vi "P4CMD_Sup Expand Wildcards.vi"(4 "string input":string) -> (1 "string output":string)   [LabVIEW 2020, in "NI_SCC_P4CMD.lvlib"]
uses:
  <vilib>/SourceControl/Providers/P4CMD/NI_SCC_P4CMD.lvlib
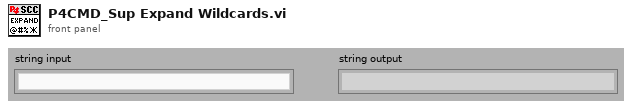
[diagram p1: front panel]
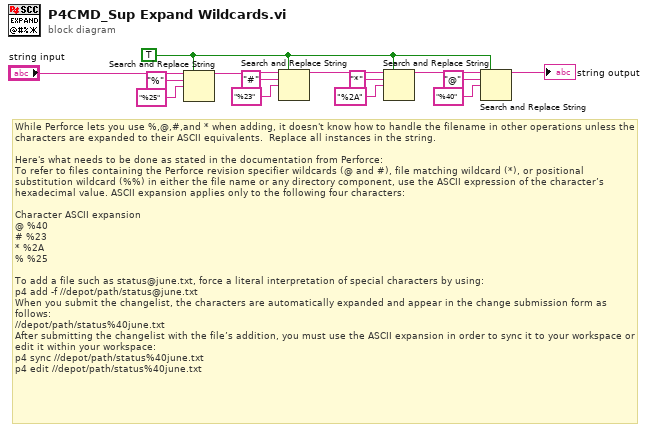
[diagram p0: block diagram]
diagram:
  w1 = TRUE ("replace all? (F)")
  # "While Perforce lets you use %,@,#,and * when adding, it doesn't know how to handle the filename in other operations unless the characters are expanded to their ASCII equivalents.  Replace all instances in the string.\n\nHere's what needs to be done as stated in the documentation from Perforce:\nTo refer to files containing the Perforce revision specifier wildcards (@ and #), file matching wildcard (*), or positional substitution wildcard (%%) in either the file name or any directory component, use the ASCII expression of the character’s hexadecimal value. ASCII expansion applies only to the following four characters:\n\nCharacter ASCII expansion\n@ %40\n# %23\n* %2A\n% %25\n\nTo add a file such as status@june.txt, force a literal interpretation of special characters by using:\np4 add -f //depot/path/status@june.txt\nWhen you submit the changelist, the characters are automatically expanded and appear in the change submission form as follows:\n//depot/path/status%40june.txt\nAfter submitting the changelist with the file’s addition, you must use the ASCII expansion in order to sync it to your workspace or edit it within your workspace:\np4 sync //depot/path/status%40june.txt\np4 edit //depot/path/status%40june.txt"
  n1 = Search and Replace String(replace all?=w1, input string="string input", search string="%", replace string="%25" ("search string")) -> (result string=w5:string)  [unwired: 4 in, 3 out]
  n2 = Search and Replace String(replace all?=w1, input string=w5, search string="#", replace string="%23" ("search string")) -> (result string=w4:string)  [unwired: 4 in, 3 out]
  n3 = Search and Replace String(replace all?=w1, input string=w4, search string="*", replace string="%2A" ("search string")) -> (result string=w3:string)  [unwired: 4 in, 3 out]
  n4 = Search and Replace String(replace all?=w1, input string=w3, search string="@", replace string="%40" ("search string")) -> (result string=→"string output":string)  [unwired: 4 in, 3 out]
